vi "CreateBufferArray.vi"() -> (0 "VI Refnum":refnum<vi>, 3 "initialized array":dbl[](array[numeric]))   [LabVIEW 2014, in "LVTiePie.lvlib"]
uses:
  LVTiePie.lvlib
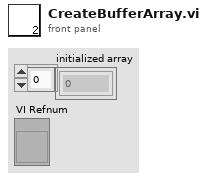
[diagram p1: front panel]
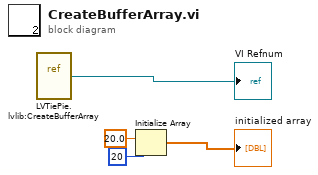
[diagram p0: block diagram]
diagram:
  n1 = vi-ref "LVTiePie.lvlib:CreateBufferArray.vi"() -> (→"VI Refnum":refnum<vi>)
  n2 = Initialize Array(20.0 ("element"), 20 ("dimension size")) -> (→"initialized array":dbl[])
